vi "Configure Counter Characteristics.vi"(0 "VISA resource name":refnum<visa-resource-name>, 1 "Counter Digits (5)":dbl=5.0, 5 "Enable Counter (F: Disable)":bool, 7 "Counter Source (0: Channel 1)":i32(ring) items=["Channel 1", "Channel 2", "Channel 3", "Channel 4", "Trigger Qualified Event"], 9 "Counter Mode (0: Frequency)":i32(ring) items=["Frequency", "Period", "Totalize"], 11 "error in (no error)":errorcluster) -> (4 "VISA resource name out":refnum<visa-resource-name>, 15 "error out":errorcluster)   [LabVIEW 2015, in "Agilent 2000 3000 X-Series.lvlib"]
doc: "Configures the counter characteristics.\n\nNote:\nThis VI is not supported by 1000 X-Series"
uses:
  Agilent 2000 3000 X-Series.lvlib
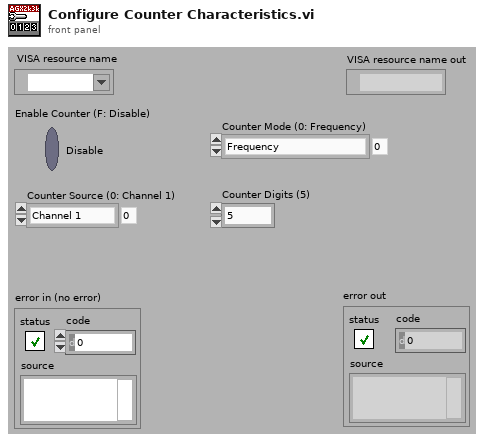
[diagram p1: front panel]
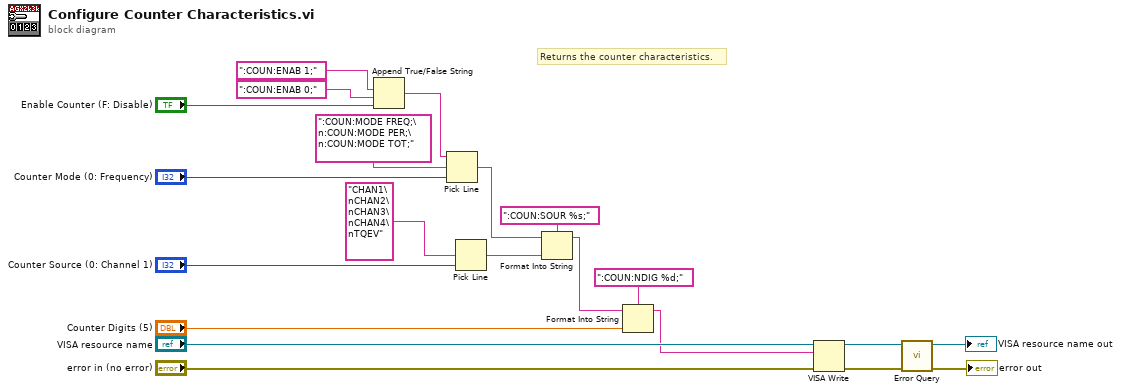
[diagram p0: block diagram]
diagram:
  # "Returns the counter characteristics."
  n1 = Append True/False String(1:"Enable Counter (F: Disable)", 2:":COUN:ENAB 0;" ("false string"), 3:":COUN:ENAB 1;" ("true string")) -> (0:w11:string)  [unwired: 1 in]
  n2 = Pick Line(string ("")=w11, multi-line string=":COUN:MODE FREQ;\n:COUN:MODE PER;\n:COUN:MODE TOT;", line index="Counter Mode (0: Frequency)") -> (output string=w8:string)
  n3 = Pick Line(multi-line string="CHAN1\nCHAN2\nCHAN3\nCHAN4\nTQEV", line index="Counter Source (0: Channel 1)") -> (output string=w5:string)  [unwired: 1 in]
  n4 = Format Into String(format string=":COUN:SOUR %s;", initial string=w8, w5) -> (resulting string=w4:string)  [unwired: 1 in, 1 out]
  n5 = Format Into String(format string=":COUN:NDIG %d;", initial string=w4, "Counter Digits (5)") -> (resulting string=w1:string)  [unwired: 1 in, 1 out]
  n6 = VISA Write(VISA resource name="VISA resource name", write buffer=w1, error in (no error)="error in (no error)") -> (VISA resource name out=w19:refnum<visa-resource-name>, error out=w18:errorcluster)  [unwired: 1 out]
  n7 = call "Error Query.vi"("error in (no error)"=w18, "VISA resource name"=w19) -> ("error out"=→"error out":errorcluster, "VISA resource name out"=→"VISA resource name out":refnum<visa-resource-name>)  [unwired: 8 out]
